vi "DSF.Engine.Pool.Plugin Interface.Create.vi"(8 "error in (no error)":errorcluster, 10 "Plugin Interfaces":refnum<class "DSF.Engine.Interface.Plugin.lvclass">[](array[class]), 11 "Plugin Interface Pool type":refnum<class "DSF.Engine.Pool.Plugin Interface.lvclass">) -> (0 "error out":errorcluster, 3 "Plugin Interface Pool out":refnum<class "DSF.Engine.Pool.Plugin Interface.lvclass">)   [LabVIEW 2016, in "DSF.Engine.lvlib" / "DSF.Engine.Pool.Plugin Interface.lvclass"]
uses:
  DSF.Engine.Pool.Plugin Interface.lvclass
  C:/Git/Sourcetree/DSF/Source/Engine/Classes/Thread Pool/DSF.Engine.Pool.lvclass
  Interface/DSF.Engine.Interface.Plugin.lvclass
  DSF.Engine.Pool.Plugin Interface.lvclass/DSF.Engine.Pool.Plugin Interface.ctl
  DSF.Engine.Pool.lvclass
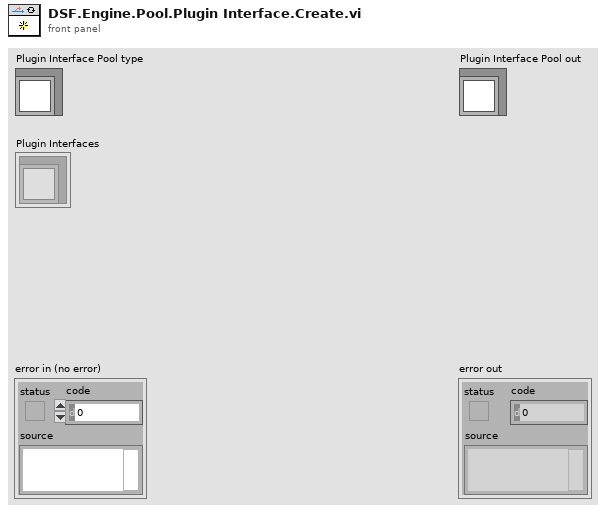
[diagram p1: front panel]
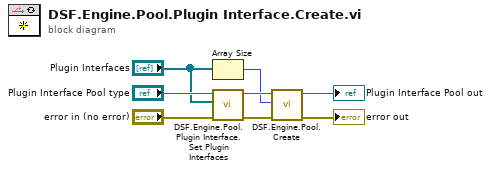
[diagram p0: block diagram]
diagram:
  n1 = Array Size(array="Plugin Interfaces") -> (size(s)=w1:i32)
  n2 = call "DSF.Engine.Pool.Plugin Interface.Set Plugin Interfaces.vi"("Plugin Interfaces"="Plugin Interfaces", "Plugin Interface Pool in"="Plugin Interface Pool type") -> ("Plugin Interface Pool out"=w4:refnum<class "DSF.Engine.Pool.Plugin Interface.lvclass">)  [unwired: 9 in]
  n3 = call "DSF.Engine.Pool.Create.vi"("error in (no error)"="error in (no error)", "number of elements"=w1, "Pool type"=w4) -> ("error out"=→"error out":errorcluster, "Pool"=→"Plugin Interface Pool out":refnum<class "DSF.Engine.Pool.Plugin Interface.lvclass">)  [unwired: 7 in]
